vi "Configure Event Search (Runt).vi"(6 "Time Threshold (2E-8 S)":dbl=2e-08, 7 "Polarity (0: Positive)":i32(ring) items=["Positive", "Negative", "Either"], 8 "error in (no error)":errorcluster, 9 "Qualifier (0: Greater)":i32(ring) items=["Greater", "Less", "None"], 10 "Source Channel (0: Channel 1)":i32(ring) items=["Channel 1", "Channel 2", "Channel 3", "Channel 4"], 11 "VISA resource name":refnum<visa-resource-name>) -> (0 "error out":errorcluster, 3 "VISA resource name out":refnum<visa-resource-name>)   [LabVIEW 2017, in "Agilent 2000 3000 X-Series.lvlib"]
doc: "Configures the event search of Runt.\n\nNotes:\nThis VI is not supported by EDUX1052A/G, DSOX1202A/G, DSOX1204A/G models."
uses:
  Agilent 2000 3000 X-Series.lvlib
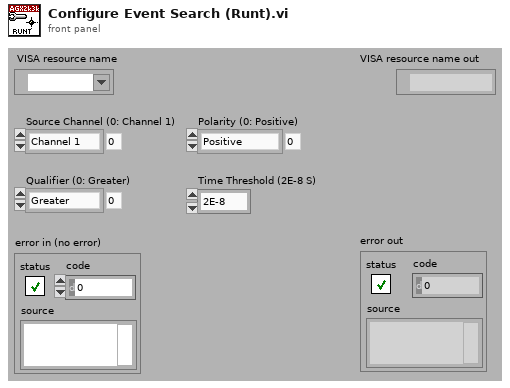
[diagram p1: front panel]
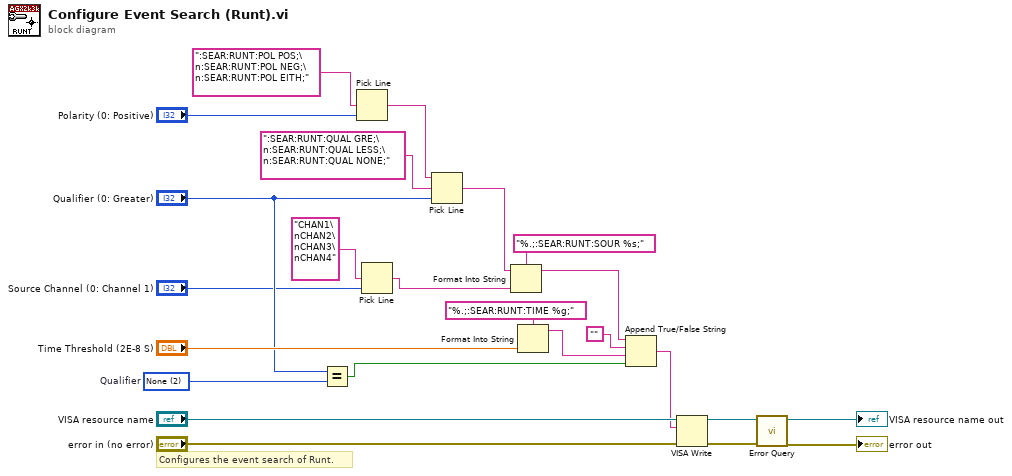
[diagram p0: block diagram]
diagram:
  w9 = 2 items=["Greater", "Less", "None"]  # Qualifier
  # "Configures the event search of Runt."
  n1 = Equal?(x="Qualifier (0: Greater)", y=w9) -> (x = y?=w8:bool)
  n2 = Pick Line(multi-line string=":SEAR:RUNT:POL POS;\n:SEAR:RUNT:POL NEG;\n:SEAR:RUNT:POL EITH;", line index="Polarity (0: Positive)") -> (output string=w21:string)  [unwired: 1 out]
  n3 = Pick Line(multi-line string="CHAN1\nCHAN2\nCHAN3\nCHAN4", line index="Source Channel (0: Channel 1)") -> (output string=w1:string)  [unwired: 1 out]
  n4 = Pick Line(string ("")=w21, multi-line string=":SEAR:RUNT:QUAL GRE;\n:SEAR:RUNT:QUAL LESS;\n:SEAR:RUNT:QUAL NONE;", line index="Qualifier (0: Greater)") -> (output string=w12:string)
  n5 = Format Into String(format string="%.;:SEAR:RUNT:SOUR %s;", initial string=w12, w1) -> (resulting string=w6:string)  [unwired: 1 in, 1 out]
  n6 = Format Into String(format string="%.;:SEAR:RUNT:TIME %g;", "Time Threshold (2E-8 S)") -> (resulting string=w7:string)  [unwired: 2 in, 1 out]
  n7 = Append True/False String(1:w8, 2:w7, 3:"", 4:w6) -> (0:w4:string)
  n8 = VISA Write(VISA resource name="VISA resource name", write buffer=w4, error in (no error)="error in (no error)") -> (VISA resource name out=w16:refnum<visa-resource-name>, error out=w15:errorcluster)  [unwired: 1 out]
  n9 = call "Error Query.vi"("error in (no error)"=w15, "VISA resource name"=w16) -> ("error out"=→"error out":errorcluster, "VISA resource name out"=→"VISA resource name out":refnum<visa-resource-name>)  [unwired: 8 out]
